vi "QCA - DUT Open NART Connection Dll.vi"(0 "NART Path":string, 5 "IP Address (\"\": localhost)":string, 7 "port (2390)":u32=2390, 12 "Timeout (2500ms)":i32=2500) -> (4 "NART TCP Connection":refnum<k5>)   [LabVIEW 2011]
panel:
  out "error_code":i32
  in  "error in (no error)":errorcluster
  out "error out":errorcluster
  in  "NART Directory":path
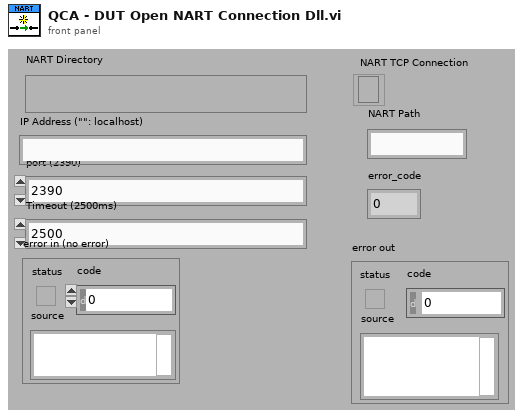
[diagram p1: front panel]
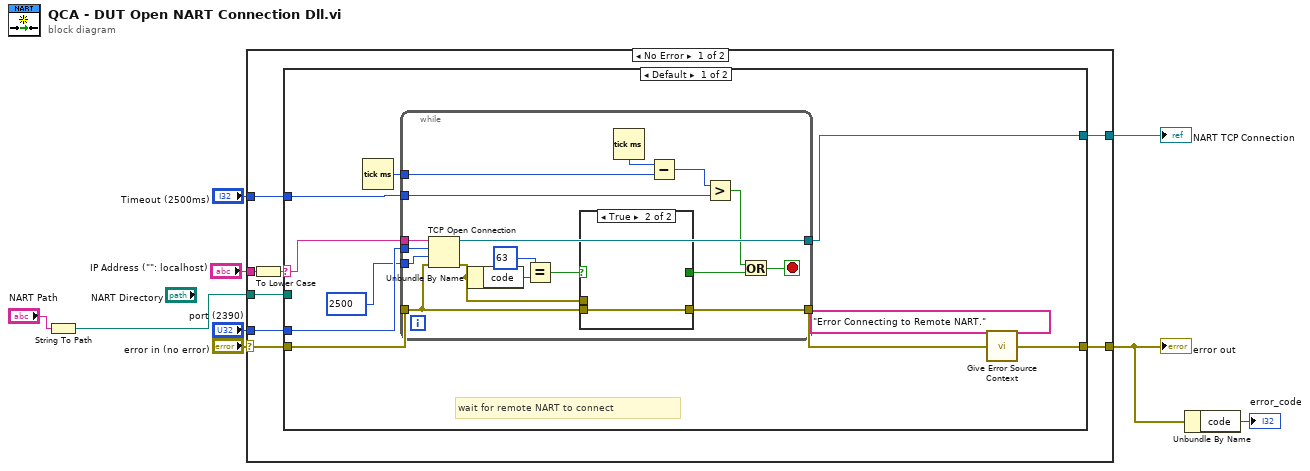
[diagram p0: block diagram]
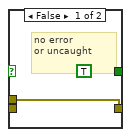
[diagram p2: hidden frame]
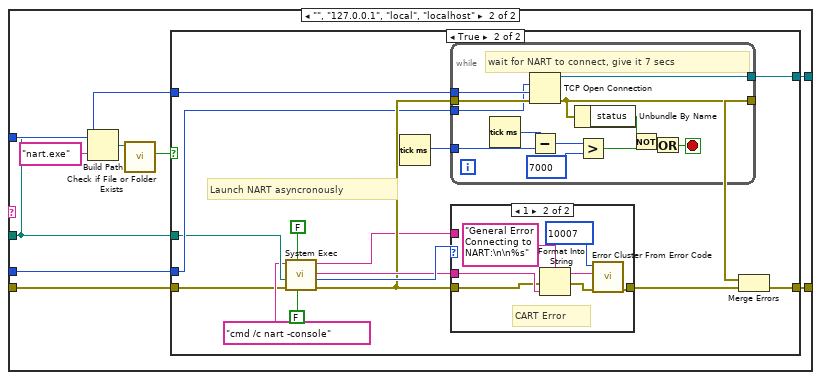
[diagram p3: hidden frame]
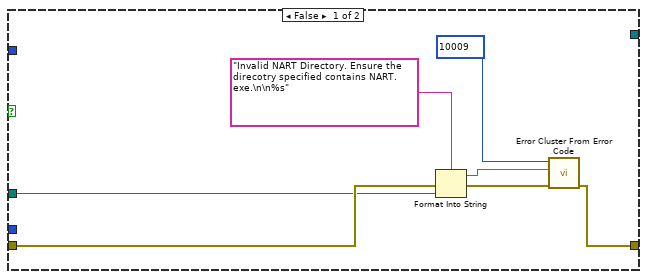
[diagram p4: hidden frame]
diagram:
  n1 = String To Path(string="NART Path") -> (path=w3:path)
  n2 = case shown="No Error" "error in (no error)" {
    selector: "error in (no error)" -> [w15 w101]
    tunnel: [w10 w101] -> w2
    tunnel: "Timeout (2500ms)" -> [w17 _]
    tunnel: [w11 _] -> w6
    tunnel: "port (2390)" -> [w16 _]
    tunnel: w3 -> [w14 _]
    tunnel: "IP Address (\"\": localhost)" -> [w13 _]
    frame No Error {
      n3 = To Lower Case(string=w13) -> (all lower case string=w12:string)
      n4 = case shown="Default" w12 {
        selector: w12 -> [w27 _]
        tunnel: [w22 w56] -> w10
        tunnel: w17 -> [w19 w55]
        tunnel: [w25 w54] -> w11
        tunnel: w16 -> [w26 w53]
        tunnel: w15 -> [w24 w52]
        tunnel: w14 -> [_ w49]
        frame Default {
          # "wait for remote NART to connect"
          n5 = Tick Count (ms)() -> (millisecond timer value=w20:u32)
          n6 = while {
            tunnel: w27 -> [w44]
            tunnel: w26 -> [w43]
            tunnel: [w42] -> w25
            tunnel: w24 -> [w37]
            tunnel: [w39] -> w23
            tunnel: w20 -> [w34]
            tunnel: w19 -> [w32]
            tunnel: 2500 ("timeout ms (60000)") -> [w28]
            stop <- w29 stop-if-true
            n7 = TCP Open Connection(address=w44, remote port or service name=w43, timeout ms (60000)=w28, error in (no error)=w37) -> (connection ID=w42:refnum<k5>, error out=w38:errorcluster)  [unwired: 1 in]
            n8 = Unbundle By Name(w38) -> ("code"=w41:i32)
            n9 = Equal?(x=63, y=w41) -> (x = y?=w36:bool)
            n10 = case shown="True" w36 {
              tunnel: [w46 w47] -> w39
              tunnel: w38 -> [w46 _]
              tunnel: [TRUE ("status") _] -> w30
              tunnel: w37 -> [_ w47]
              frame False {
                # "no error\nor uncaught"
              }
              frame True {
              }
            }
            n11 = Tick Count (ms)() -> (millisecond timer value=w35:u32)
            n12 = Subtract(x=w35, y=w34) -> (x-y=w33:u32)
            n13 = Greater?(x=w33, y=w32) -> (0:w31:bool)
            n14 = Or(x=w31, y=w30) -> (x .or. y?=w29:bool)
          }
          n15 = call "Give Error Source Context.vi"("Context String"="Error Connecting to Remote NART." ("string"), "error in"=w23) -> ("Error out with context"=w22:errorcluster)  [unwired: 13 in]
        }
        frame "", "127.0.0.1", "local", "localhost" {
          n16 = Build Path(base path=w49, name or relative path="nart.exe") -> (appended path=w50:path)
          n17 = call <vilib>:"Check if File or Folder Exists.vi"("path"=w50) -> ("file or folder exists?"=w48:bool)  [unwired: 8 in, 2 out]
          n18 = case shown="True" w48 {
            tunnel: [w59 w79] -> w56
            tunnel: w55 -> [_ w78]
            tunnel: [_ w77] -> w54
            tunnel: w53 -> [_ w69]
            tunnel: w52 -> [w58 w64]
            tunnel: w49 -> [w57 w66]
            frame False {
              n19 = Format Into String(format string="Invalid NART Directory. Ensure the direcotry specified contains NART.exe.\n\n%s", error in=w58, w57) -> (resulting string=w62:string, error out=w60:errorcluster)  [unwired: 1 in]
              n20 = call <vilib>:"Error Cluster From Error Code.vi"("error in (no error)"=w60, "error message (\"\")"=w62, "error code (0)"=10009) -> ("error out"=w59:errorcluster)  [unwired: 6 in]
            }
            frame True {
              # "Launch NART asyncronously"
              n21 = call <vilib>:"System Exec.vi"("run minimized? (F)"=FALSE, "wait until completion? (T)"=FALSE, "error in (no error)"=w64, "working directory"=w66, "command line"="cmd /c nart -console" ("format string")) -> ("error out"=w70:errorcluster, "return code"=w75:i32, "standard error"=w73:string, "standard output"=w68:string)  [unwired: 3 in]
              n22 = Tick Count (ms)() -> (millisecond timer value=w67:u32)
              n23 = while {
                tunnel: w78 -> [w92]
                tunnel: [w91] -> w77
                tunnel: [w84] -> w76
                tunnel: w70 -> [w90]
                tunnel: w69 -> [w89]
                tunnel: w67 -> [w87]
                stop <- w83 stop-if-true
                # "wait for NART to connect, give it 7 secs"
                n24 = Tick Count (ms)() -> (millisecond timer value=w88:u32)
                n25 = TCP Open Connection(remote port or service name=w89, timeout ms (60000)=w92, error in (no error)=w90) -> (connection ID=w91:refnum<k5>, error out=w84:errorcluster)  [unwired: 2 in]
                n26 = Subtract(x=w88, y=w87) -> (x-y=w86:u32)
                n27 = Unbundle By Name(w84) -> ("status"=w81:bool)
                n28 = Greater?(x=w86, y=u32 7000) -> (0:w82:bool)
                n29 = Not(x=w81) -> (.not. x?=w80:bool)
                n30 = Or(x=w80, y=w82) -> (x .or. y?=w83:bool)
              }
              n31 = case shown="1" w75 {
                tunnel: w70 -> [w93 w95]
                tunnel: [w93 w100] -> w74
                tunnel: w73 -> [_ w96]
                tunnel: w68 -> [_ _]
                frame Default {
                }
                frame 1 {
                  # "CART Error"
                  n32 = Format Into String(format string="General Error Connecting to NART:\n\n%s", error in=w95, w96) -> (resulting string=w98:string, error out=w94:errorcluster)  [unwired: 1 in]
                  n33 = call <vilib>:"Error Cluster From Error Code.vi"("error in (no error)"=w94, "error message (\"\")"=w98, "error code (0)"=10007) -> ("error out"=w100:errorcluster)  [unwired: 6 in]
                }
              }
              n34 = Merge Errors(w76, w74) -> (w79:errorcluster)
            }
          }
        }
      }
    }
    frame Error {
    }
  }
  "error out" <- w2
  "NART TCP Connection" <- w6
  n35 = Unbundle By Name(w2) -> ("code"=→"error_code":i32)
